vi "Network Send.vi"(8 "error in (no error)":errorcluster, 11 "Electrophysiology in":refnum<class "Electrophysiology.lvclass">) -> (0 "error out":errorcluster, 2 "Connected":bool, 3 "Electrophysiology out":refnum<class "Electrophysiology.lvclass">)   [LabVIEW 2014, in "Electrophysiology.lvclass"]
uses:
  Electrophysiology.lvclass
  Electrophysiology.lvclass/Electrophysiology.ctl
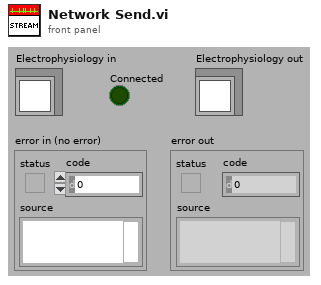
[diagram p1: front panel]
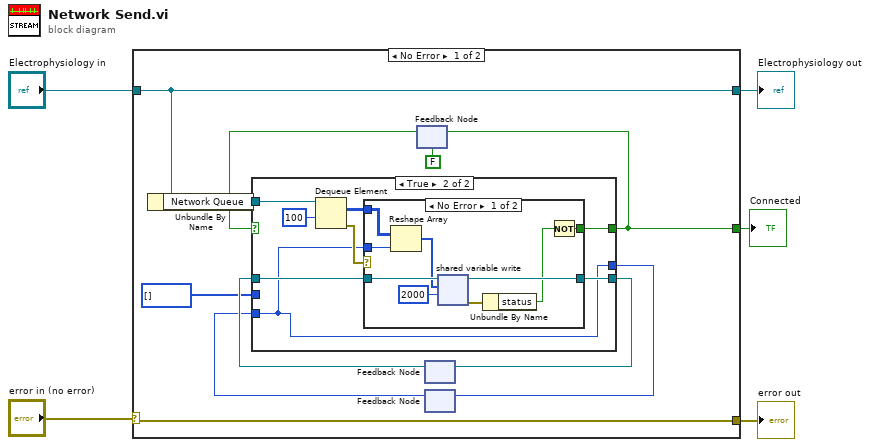
[diagram p0: block diagram]
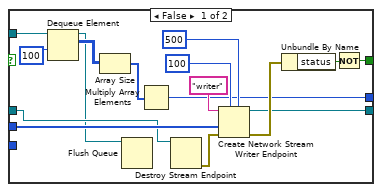
[diagram p2: hidden frame]
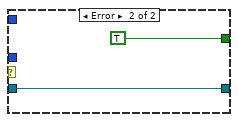
[diagram p3: hidden frame]
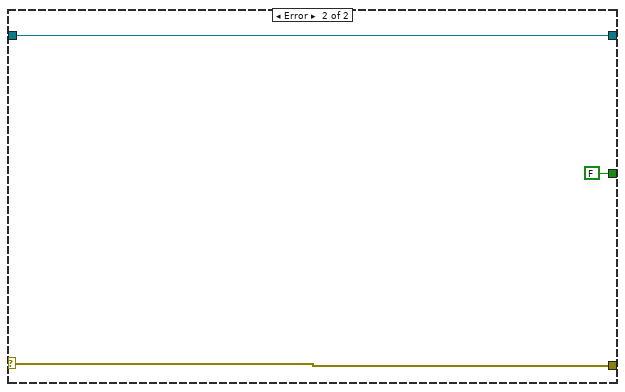
[diagram p4: hidden frame]
diagram:
  n1 = case shown="No Error" "error in (no error)" {
    selector: "error in (no error)" -> [w16 w54]
    tunnel: [w16 w54] -> w4
    tunnel: [w10 w53] -> w2
    tunnel: "Electrophysiology in" -> [w10 w53]
    tunnel: [w6 FALSE] -> w1
    frame No Error {
      n2 = Unbundle By Name(w10) -> ("Network Queue"=w9:refnum<queue>)
      n3 = feedback #1(FALSE) -> (w15:bool)
      n4 = feedback #2() -> (w13:refnum<k21>)  [unwired: 1 in]
      n5 = feedback #3() -> (w7:i32)  [unwired: 1 in]
      n6 = case shown="True" w15 {
        tunnel: i32[] [] -> [w29 _]
        tunnel: [w25 w34] -> w6
        tunnel: [w27 w37] -> w14
        tunnel: w13 -> [w24 w39]
        tunnel: w9 -> [w21 w40]
        tunnel: [w17 w33] -> w8
        tunnel: w7 -> [_ w33]
        frame False {
          n7 = Dequeue Element(queue=w21, timeout in ms (-1)=100) -> (queue out=w19:refnum<queue>, element=w20:i32[][])  [unwired: 1 in, 2 out]
          n8 = Array Size(array=w20) -> (size(s)=w18:i32[])
          n9 = Flush Queue(queue=w19) -> ()  [unwired: 1 in, 3 out]
          n10 = Multiply Array Elements(1:w18) -> (0:w17:i32)
          n11 = Destroy Stream Endpoint(11:w24) -> (0:w23:errorcluster)  [unwired: 1 in]
          n12 = Create Network Stream Writer Endpoint(5:500 ("timeout in ms (-1)"), 7:100 ("writer buffer size"), 8:w23, 9:w29, 11:"writer" ("writer name")) -> (0:w28:errorcluster, 3:w27:refnum<k21>)  [unwired: 2 in]
          n13 = Unbundle By Name(w28) -> ("status"=w26:bool)
          n14 = Not(x=w26) -> (.not. x?=w25:bool)
        }
        frame True {
          n15 = Dequeue Element(queue=w40, timeout in ms (-1)=100) -> (element=w38:i32[][], error out=w35:errorcluster)  [unwired: 1 in, 2 out]
          n16 = case shown="No Error" w35 {
            tunnel: w39 -> [w49 w51]
            tunnel: w38 -> [w44 _]
            tunnel: [w48 w51] -> w37
            tunnel: [w45 TRUE] -> w34
            tunnel: w33 -> [w43 _]
            frame No Error {
              n17 = Reshape Array(w44, w43) -> (w42:i32[])
              n18 = shared-variable-write(w49, w42, 2000 ("timeout ms (-1)")) -> (w48:refnum<k21>, w47:errorcluster)  [unwired: 1 in, 1 out]
              n19 = Unbundle By Name(w47) -> ("status"=w46:bool)
              n20 = Not(x=w46) -> (.not. x?=w45:bool)
            }
            frame Error {
            }
          }
        }
      }
      n21 = feedback-in #1(w6) -> ()
      n22 = feedback-in #2(w14) -> ()
      n23 = feedback-in #3(w8) -> ()
    }
    frame Error {
    }
  }
  "error out" <- w4
  "Electrophysiology out" <- w2
  "Connected" <- w1
